vi "GoBang_CheckLine.vi"(0 "line with 5 elements":u8[](array[numeric])=[0, 0, 0, 0, 0]) -> (1 "White won":bool, 2 "Black won":bool)   [LabVIEW 2013, in "GoBang.lvlib"]
uses:
  GoBang.lvlib
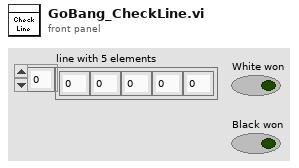
[diagram p1: front panel]
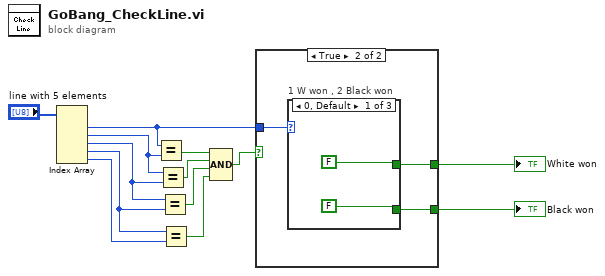
[diagram p0: block diagram]
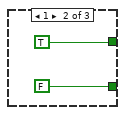
[diagram p3: hidden frame]
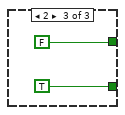
[diagram p4: hidden frame]
diagram:
  n1 = Index Array(array="line with 5 elements") -> (element #1=w10:u8, element #2=w9:u8, element #3=w8:u8, element #4=w7:u8, element #5=w6:u8)  [unwired: 5 in]
  n2 = Equal?(x=w10, y=w9) -> (x = y?=w5:bool)
  n3 = Equal?(x=w9, y=w8) -> (x = y?=w4:bool)
  n4 = Equal?(x=w8, y=w7) -> (x = y?=w3:bool)
  n5 = Equal?(x=w7, y=w6) -> (x = y?=w2:bool)
  n6 = Compound Arithmetic op=AND(w5, w4, w3, w2) -> (w1:bool)
  n7 = case shown="True" w1 {
    tunnel: [_ w16] -> w13
    tunnel: [_ w15] -> w12
    tunnel: w10 -> [_ w14]
    frame False {
    }
    frame True {
      n8 = case "1 W won , 2 Black won" shown="0, Default" w14 {
        tunnel: [FALSE TRUE FALSE] -> w16
        tunnel: [FALSE FALSE TRUE] -> w15
        frame 0, Default {
        }
        frame 1 {
        }
        frame 2 {
        }
      }
    }
  }
  "Black won" <- w12
  "White won" <- w13
